vi "Click Array.vi"(10 "Coords":T1, 11 "CtlRef":refnum<vi>) -> (0 "error out":errorcluster, 2 "Open?":bool, 3 "SR Number":i32)   [LabVIEW 2018]
uses:
  <vilib>/Utility/miscctls.llb/LVPoint32TypeDef.ctl
  Type Defs/SR Cluster.ctl
  Type Defs/SR Status.ctl
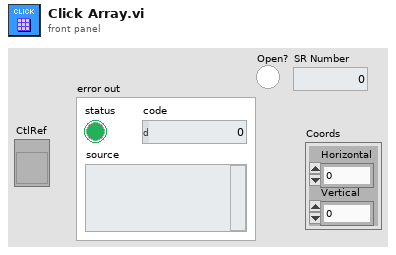
[diagram p1: front panel]
types:
  T1 = typedef "LVPoint32TypeDef.ctl" = cluster{"Horizontal":i32, "Vertical":i32}
  T2 = typedef "SR Cluster.ctl" = cluster{"Color":u32, "SR Number":i32, "SR Status":T3, "Name":string, "Summary":string, "Last Updated":timestamp, "SR Type":string, "Service Level":string, "Days Open":dbl, "Creation Date":timestamp, "Owner":string, "Note":string}
  T3 = typedef "SR Status.ctl" = enum16{"Caller Abandoned", "Created in Error", "Expired", "Forum Resolved AE", "Forum Resolved Customer", "IN WORK", "IN WORK Collab with AES", "IN WORK Collab with PSE", "IN WORK Collab with SE", "IN WORK Customer Added Note", "IN WORK Escalation", "IN WORK Wait on Customer", "Open", "Potentially Resolved", "Presumed Resolved", "RMA Approved for Return", "RMA Closed", "RMA Closed - DOA", "RMA In Progress", "RMA Open", "RMA Waiting on Customer", "Resolved", "Passed Off"}
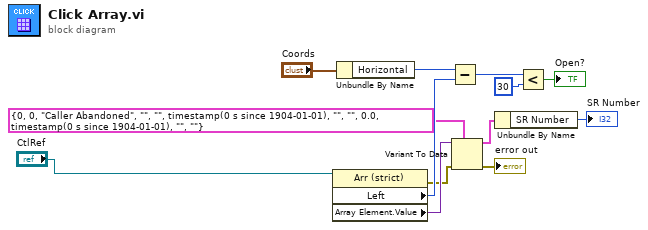
[diagram p0: block diagram]
diagram:
  n1 = property class="Arr (strict)"(reference="CtlRef") -> (error out=w4:errorcluster, "Left"=w12:i32, "Array Element.Value"=w6:variant)  [unwired: 1 in, 1 out]
  n2 = Unbundle By Name("Coords") -> ("Horizontal"=w11:i32)
  n3 = Subtract(x=w11, y=w12) -> (x-y=w10:i32)
  n4 = Variant To Data(error in=w4, type=T2 {"Color"=0, "SR Number"=0, "SR Status"=enum."Caller Abandoned", "Name"="", "Summary"="", "Last Updated"=timestamp(0 s since 1904-01-01), "SR Type"="", "Service Level"="", "Days Open"=0.0, "Creation Date"=timestamp(0 s since 1904-01-01), "Owner"="", "Note"=""} ("SR Cluster"), Variant=w6) -> (data=w5:T2, error out=→"error out":errorcluster)
  n5 = Unbundle By Name(w5) -> ("SR Number"=→"SR Number":i32)
  n6 = Less?(x=w10, y=30) -> (x < y?=→"Open?":bool)
